vi "XIPIN_Utility_Reduced_Logic_2_0.vi"   [LabVIEW 2017]
doc: "Performs logic operations on a n-bit input to produce a one bit output\n------------------------------------\n<b>Need License</b> : No"
uses:
  <vilib>/rvi/XilinxIP/XIPIN_XNode/niFpgaXIPIN.xnode
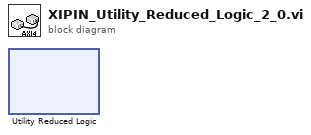
[diagram p0: block diagram]
diagram:
  n1 = xnode ("Utility Reduced Logic")() -> ()
